vi "Initialize Modbus Connection.vi"(8 "error in (no error)":errorcluster, 11 "Parameters":T1 {"Interface Data"."Serial Settings"."parity (even)" items=["None", "Odd", "Even", "Mark", "Space"]; "Interface Data"."Serial Settings"."flow control (none)" items=["None", "XON/XOFF", "RTS/CTS", "XON/XOFF & RTS/CTS", "DTR/DSR", "XON/XOFF & DTR/DSR"]}) -> (0 "error out":errorcluster, 3 "Modbus Master out":refnum<class "Modbus Master.lvclass">)   [LabVIEW 2015, in "Modbus Master Engine.lvlib"]
uses:
  Modbus Master Engine.lvlib
  Shared/Device Info.ctl
  Shared/Controls/Interface Type.ctl
  Shared/Controls/Data Model/TCP Settings.ctl
  Shared/Controls/Data Model/Serial Settings.ctl
  Bulk Data Access.ctl
  System Explorer/SubVIs/Modbus Type.ctl
  Shared/Controls/Data Model/Channel.ctl
  <vilib>/NI Veristand/Custom Device API/Custom Device Channel Type.ctl
  Shared/Controls/Data Model/Mapping.ctl
  Shared/Controls/Data Model/DataType.ctl
  <vilib>/NI Veristand/Custom Device API/Custom Device Item Ref.ctl
  Modbus API.lvlibp/API/Master/Modbus Master.lvclass
  Modbus API.lvlibp/API/Wrapper/API Main.lvlib
  Shared/Modbus Master Shared.lvlib
  <vilib>/NI VeriStand/Custom Device API/Custom Device API.lvlib
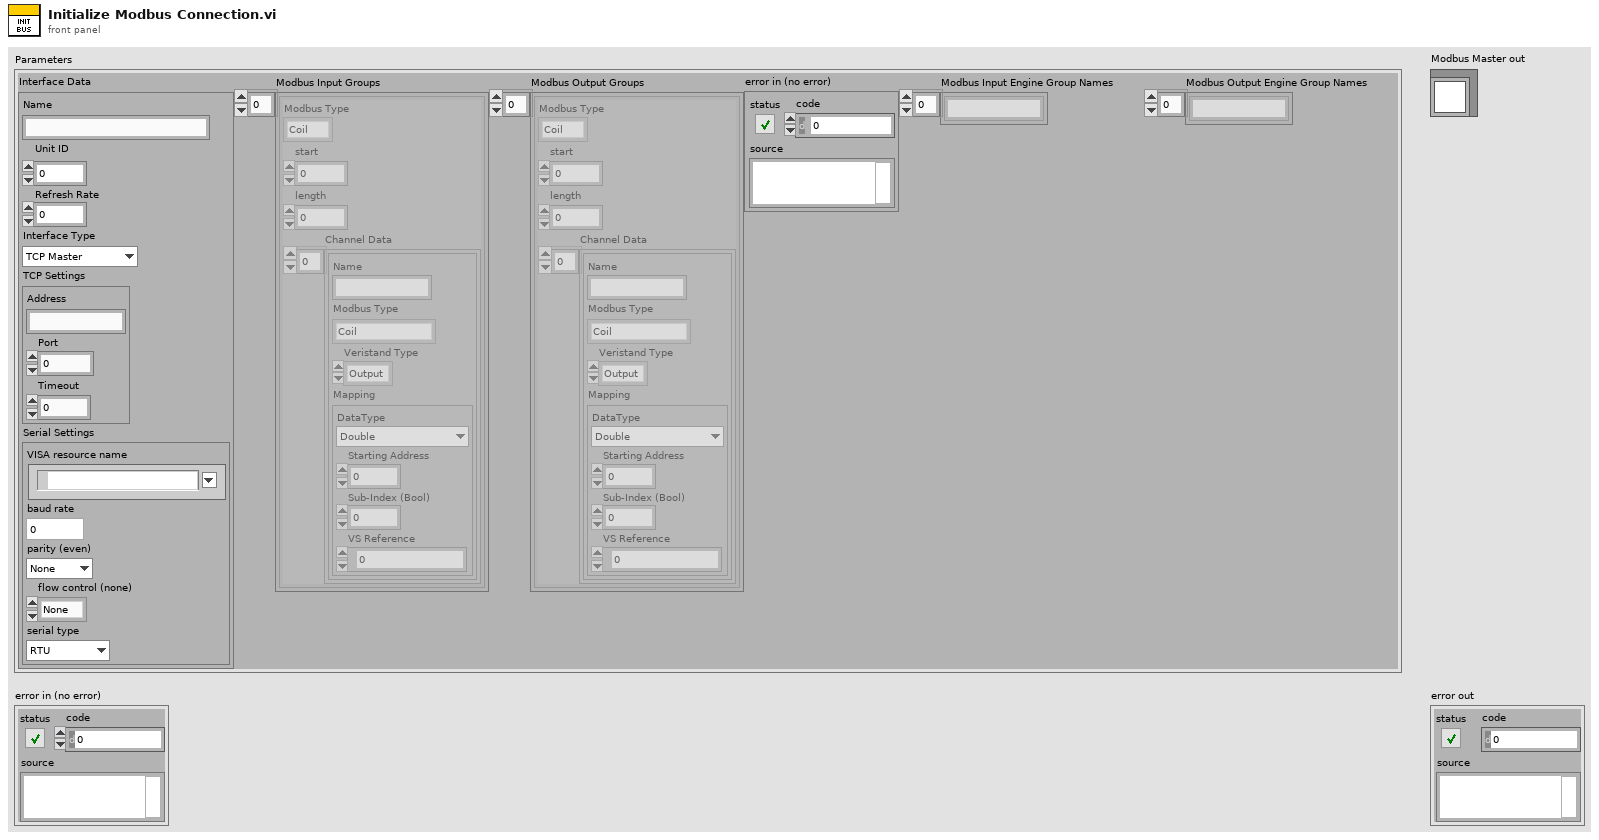
[diagram p1: front panel]
types:
  T1 = typedef "Modbus Master Shared.lvlib/Device Info.ctl" = cluster{"Interface Data":cluster{"Name":string, "Unit ID":u8, "Refresh Rate":i32, "Interface Type":T2, "TCP Settings":T3, "Serial Settings":T4}, "Modbus Input Groups":T5[], "Modbus Output Groups":T5[], "error in (no error)":errorcluster, "Modbus Input Engine Group Names":string[], "Modbus Output Engine Group Names":string[]}
  T2 = typedef "Modbus Master Shared.lvlib/Interface Type.ctl" = enum16{"TCP Master", "Serial Master"}
  T3 = typedef "Modbus Master Shared.lvlib/TCP Settings.ctl" = cluster{"Address":string, "Port":u16, "Timeout":i32}
  T4 = typedef "Modbus Master Shared.lvlib/Serial Settings.ctl" = cluster{"VISA resource name":refnum<visa-resource-name>, "baud rate":u32, "parity (even)":u16, "flow control (none)":u16, "serial type":enum16{"RTU", "ASCII"}}
  T5 = typedef "Modbus Master Shared.lvlib/Bulk Data Access.ctl" = cluster{"Modbus Type":T6, "start":u16, "length":u16, "Channel Data":T7[]}
  T6 = typedef "Modbus Master Shared.lvlib/Modbus Type.ctl" = enum16{"Coil", "Discrete Input", "Holding Register", "Input Register"}
  T7 = typedef "Modbus Master Shared.lvlib/Channel.ctl" = cluster{"Name":string, "Modbus Type":T6, "Veristand Type":T8, "Mapping":T9}
  T8 = typedef "Custom Device API.lvlib/Custom Device Channel Type.ctl" = enum16{"Input", "Output"}
  T9 = typedef "Modbus Master Shared.lvlib/Mapping.ctl" = cluster{"DataType":T10, "Starting Address":u16, "Sub-Index (Bool)":u16, "VS Reference":T11}
  T10 = typedef "Modbus Master Shared.lvlib/DataType.ctl" = enum16{"Double", "Single", "I64", "I32", "I16", "I8", "U64", "U32", "U16", "U8", "Boolean"}
  T11 = typedef "Custom Device API.lvlib/Custom Device Item Ref.ctl" = u64
  T12 = cluster{"serial master instances":refnum<class "Modbus Master.lvclass">[], "VISA Resources":refnum<visa-resource-name>[]}
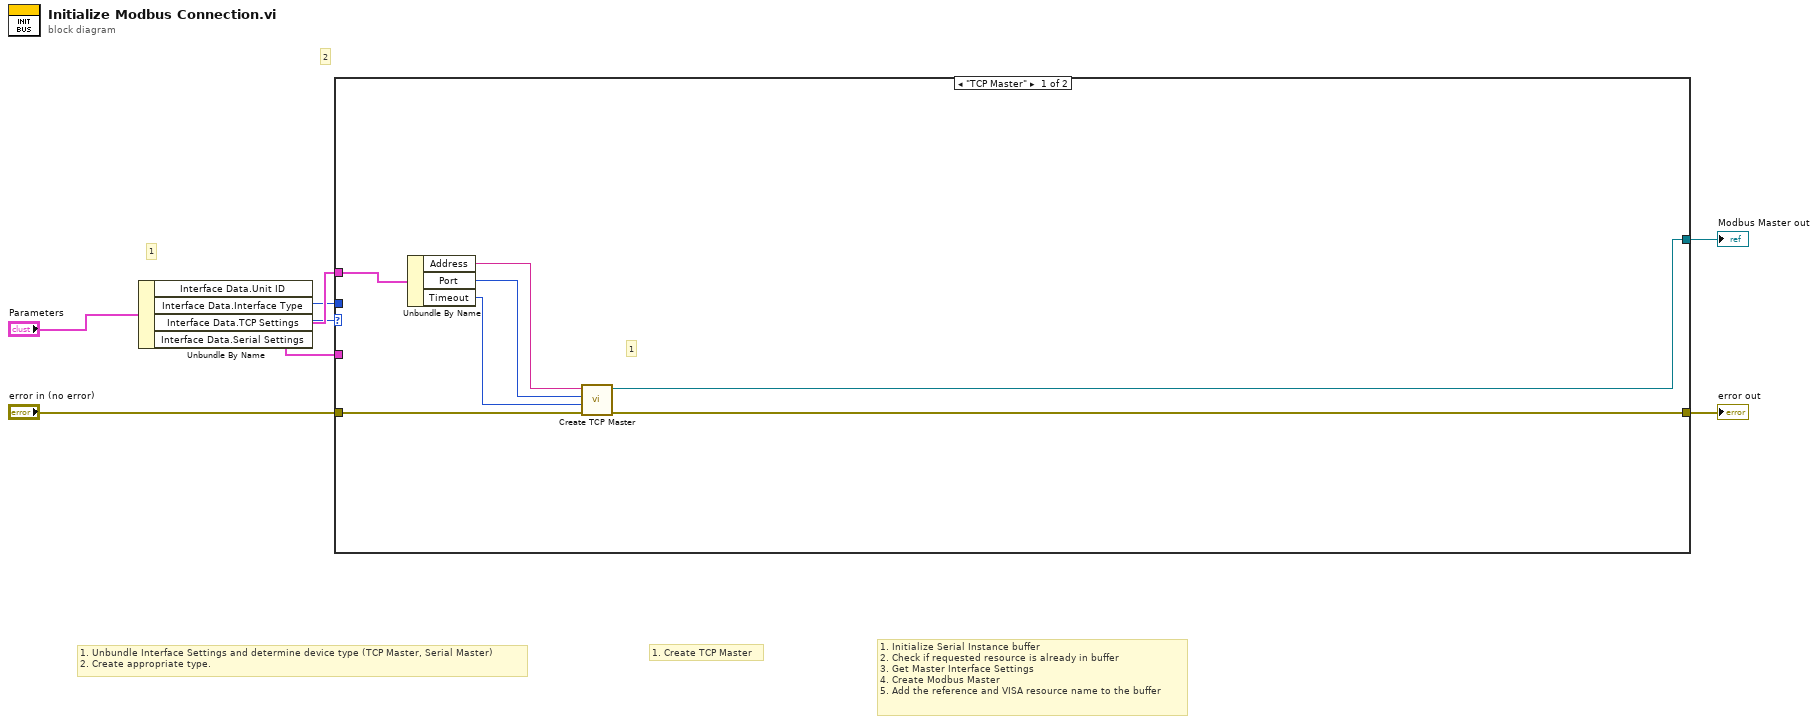
[diagram p0: block diagram]
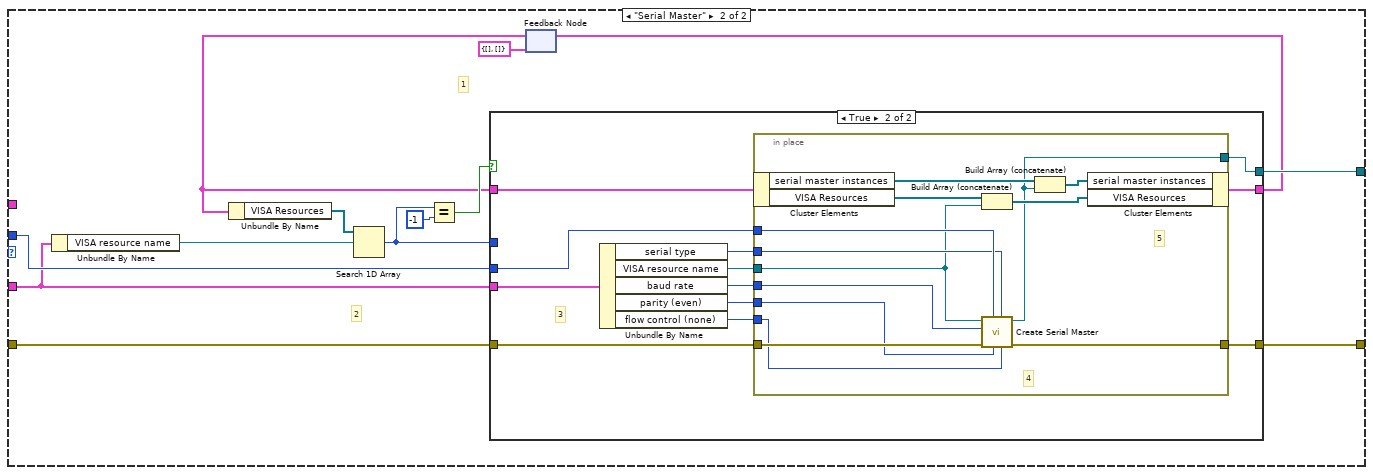
[diagram p2: hidden frame]
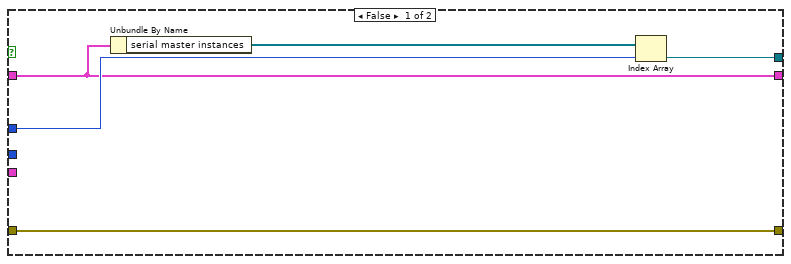
[diagram p3: hidden frame]
diagram:
  # "1. Initialize Serial Instance buffer\n2. Check if requested resource is already in buffer\n3. Get Master Interface Settings\n4. Create Modbus Master\n5. Add the reference and VISA resource name to the buffer"
  # "1. Create TCP Master"
  # "2"
  # "1"
  # "1. Unbundle Interface Settings and determine device type (TCP Master, Serial Master)\n2. Create appropriate type."
  n1 = Unbundle By Name("Parameters") -> ("Interface Data.Unit ID"=w5:u8, "Interface Data.Interface Type"=w6:T2, "Interface Data.TCP Settings"=w7:T3, "Interface Data.Serial Settings"=w8:T4)
  n2 = case shown="\"TCP Master\"" w6 {
    tunnel: w5 -> [_ w28]
    tunnel: w7 -> [w15 _]
    tunnel: w8 -> [_ w16]
    tunnel: [w12 w25] -> w1
    tunnel: [w11 w27] -> w3
    tunnel: "error in (no error)" -> [w10 w26]
    frame "TCP Master" {
      # "1"
      n3 = Unbundle By Name(w15) -> ("Address"=w14:string, "Port"=w13:u16, "Timeout"=w9:i32)
      n4 = call "Create TCP Master.vi"("error in"=w10, "connect timeout ms"=w9, "port (502)"=w13, "address"=w14) -> ("error out"=w11:errorcluster, "TCP master instance"=w12:refnum<class "Modbus Master.lvclass">)  [unwired: 6 in]
    }
    frame "Serial Master" {
      # "2"
      # "1"
      n5 = Unbundle By Name(w16) -> ("VISA resource name"=w24:refnum<visa-resource-name>)
      n6 = feedback #1(T12 {"serial master instances"=[], "VISA Resources"=[]}) -> (w19:T12)
      n7 = Unbundle By Name(w19) -> ("VISA Resources"=w18:refnum<visa-resource-name>[])
      n8 = Search 1D Array(1D array=w18, element=w24) -> (index of element=w21:i32)  [unwired: 1 in]
      n9 = Equal?(x=w21, y=-1) -> (x = y?=w22:bool)
      n10 = case shown="True" w22 {
        tunnel: w28 -> [_ w45]
        tunnel: [w32 w44] -> w27
        tunnel: w26 -> [w32 w43]
        tunnel: [w30 w42] -> w25
        tunnel: w21 -> [w33 _]
        tunnel: w19 -> [w29 w41]
        tunnel: [w29 w40] -> w17
        tunnel: w16 -> [_ w39]
        frame False {
          n11 = Unbundle By Name(w29) -> ("serial master instances"=w31:refnum<class "Modbus Master.lvclass">[])
          n12 = Index Array(array=w31, index=w33) -> (element=w30:refnum<class "Modbus Master.lvclass">)
        }
        frame True {
          # "3"
          n13 = Unbundle By Name(w39) -> ("serial type"=w38:enum16{"RTU", "ASCII"}, "VISA resource name"=w37:refnum<visa-resource-name>, "baud rate"=w36:u32, "parity (even)"=w35:u16, "flow control (none)"=w34:u16)
          n14 = in-place {
            in-place-border: w45 -> [w58]
            in-place-border: [w57] -> w44
            in-place-border: w43 -> [w56]
            in-place-border: [w46] -> w42
            in-place-border: w38 -> [w51]
            in-place-border: w37 -> [w50]
            in-place-border: w36 -> [w49]
            in-place-border: w35 -> [w48]
            in-place-border: w34 -> [w47]
            # "5"
            # "4"
            n15 = in-place-cluster #2(w41) -> ("serial master instances"=w53:refnum<class "Modbus Master.lvclass">[], "VISA Resources"=w55:refnum<visa-resource-name>[])
            n16 = Build Array (concatenate)(w55, w50) -> (w54:refnum<visa-resource-name>[])
            n17 = call "Create Serial Master.vi"("flow control (none)"=w47, "serial type"=w51, "parity (even)"=w48, "unit ID"=w58, "error in"=w56, "baud rate"=w49, "VISA resource name"=w50) -> ("error out"=w57:errorcluster, "serial master instance"=w46:refnum<class "Modbus Master.lvclass">)  [unwired: 3 in]
            n18 = Build Array (concatenate)(w53, w46) -> (w52:refnum<class "Modbus Master.lvclass">[])
            n19 = in-place-cluster #2("serial master instances"=w52, "VISA Resources"=w54) -> (w40:T12)
          }
        }
      }
      n20 = feedback-in #1(w17) -> ()
    }
  }
  "error out" <- w3
  "Modbus Master out" <- w1
